vi "BRig_dataBlock_DAB_nReward_HighProb.vi"() -> (2 "output_DAB_nReward_HighProb":i32)   [LabVIEW 2014]
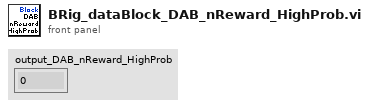
[diagram p1: front panel]
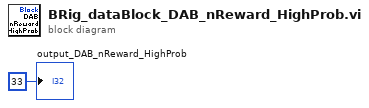
[diagram p0: block diagram]
diagram:
  "output_DAB_nReward_HighProb" <- 33 ("output_iBlock")
